vi "总磷总氮公式读取.vi"(8 "error in (no error)":errorcluster caption="错误输入（无错误）", 9 "量程":enum16{"低量程", "高量程"}(ring), 10 "测量模式":enum16{"水样测量", "零点核查", "跨度核查", "标样核查", "加标回收"}(ring), 11 "测量参数":enum16{"COD", "氨氮", "总氮", "总磷"}(ring)) -> (0 "error out":errorcluster caption="错误输出", 3 "公式":cluster{"X^2":dbl, "X":dbl, "b":dbl})   [LabVIEW 2016, in "斯坦道总氮.lvlib"]
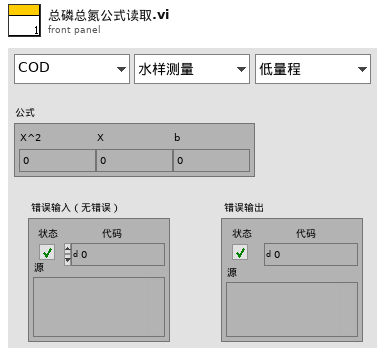
[diagram p1: front panel]
types:
  T1 = cluster{"FLOAT[0]":sgl, "FLOAT[1]":sgl, "FLOAT[2]":sgl}
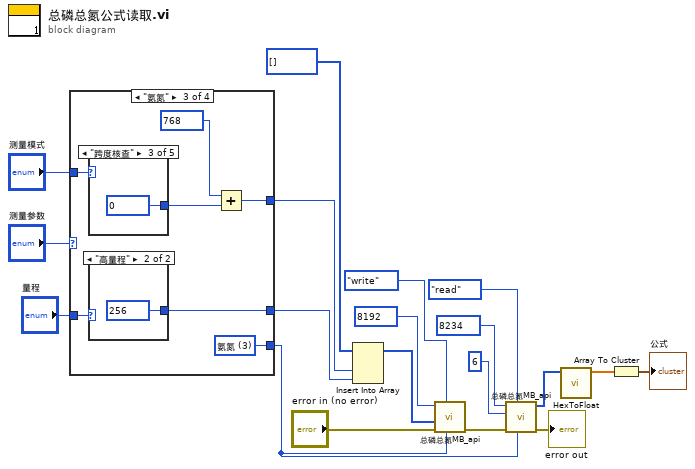
[diagram p0: block diagram]
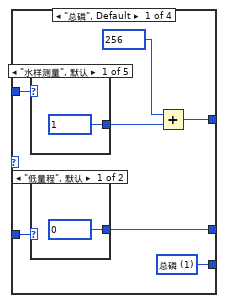
[diagram p2: hidden frame]
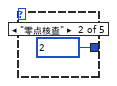
[diagram p3: hidden frame]
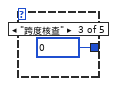
[diagram p4: hidden frame]
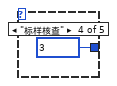
[diagram p5: hidden frame]
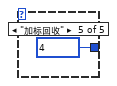
[diagram p6: hidden frame]
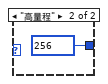
[diagram p7: hidden frame]
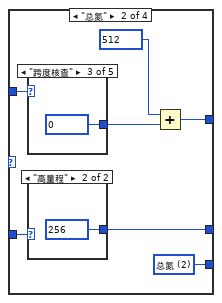
[diagram p8: hidden frame]
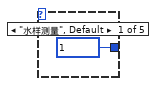
[diagram p9: hidden frame]
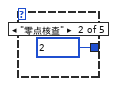
[diagram p10: hidden frame]
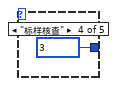
[diagram p11: hidden frame]
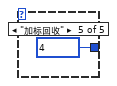
[diagram p12: hidden frame]
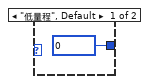
[diagram p13: hidden frame]
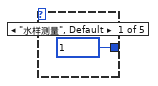
[diagram p14: hidden frame]
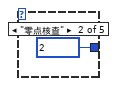
[diagram p15: hidden frame]
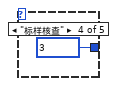
[diagram p16: hidden frame]
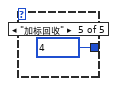
[diagram p17: hidden frame]
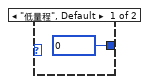
[diagram p18: hidden frame]
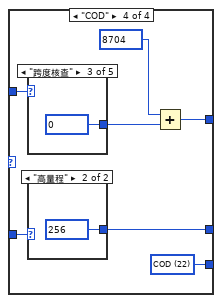
[diagram p19: hidden frame]
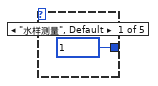
[diagram p20: hidden frame]
diagram:
  n1 = case shown="\"氨氮\"" "测量参数" {
    tunnel: "测量模式" -> [w24 w39 w53 w67]
    tunnel: "量程" -> [w25 w40 w54 w68]
    tunnel: [w26 w34 w48 w62] -> w5
    tunnel: [w20 w35 w49 w63] -> w9
    tunnel: [w23 w38 w52 w66] -> w8
    frame "总磷", Default {
      w26 = u16 1 items=["总磷"=1, "总氮"=2, "氨氮"=3] ("站号")
      n2 = case shown="\"水样测量\", 默认" w24 {
        tunnel: [u16 1 ("starting address") u16 2 ("starting address") u16 0 ("starting address") u16 3 ("starting address") u16 4 ("starting address")] -> w22
        frame "水样测量", Default {
        }
        frame "零点核查" {
        }
        frame "跨度核查" {
        }
        frame "标样核查" {
        }
        frame "加标回收" {
        }
      }
      n3 = case shown="\"低量程\", 默认" w25 {
        tunnel: [u16 0 ("starting address") u16 256 ("starting address")] -> w23
        frame "低量程", Default {
        }
        frame "高量程" {
        }
      }
      n4 = Add(x=u16 256 ("starting address"), y=w22) -> (x+y=w20:u16)
    }
    frame "总氮" {
      w34 = u16 2 items=["总磷"=1, "总氮"=2, "氨氮"=3] ("站号")
      n5 = case shown="\"跨度核查\"" w39 {
        tunnel: [u16 1 ("starting address") u16 2 ("starting address") u16 0 ("starting address") u16 3 ("starting address") u16 4 ("starting address")] -> w37
        frame "水样测量", Default {
        }
        frame "零点核查" {
        }
        frame "跨度核查" {
        }
        frame "标样核查" {
        }
        frame "加标回收" {
        }
      }
      n6 = case shown="\"高量程\"" w40 {
        tunnel: [u16 0 ("starting address") u16 256 ("starting address")] -> w38
        frame "低量程", Default {
        }
        frame "高量程" {
        }
      }
      n7 = Add(x=u16 512 ("starting address"), y=w37) -> (x+y=w35:u16)
    }
    frame "氨氮" {
      w48 = u16 3 items=["总磷"=1, "总氮"=2, "氨氮"=3] ("站号")
      n8 = case shown="\"跨度核查\"" w53 {
        tunnel: [u16 1 ("starting address") u16 2 ("starting address") u16 0 ("starting address") u16 3 ("starting address") u16 4 ("starting address")] -> w51
        frame "水样测量", Default {
        }
        frame "零点核查" {
        }
        frame "跨度核查" {
        }
        frame "标样核查" {
        }
        frame "加标回收" {
        }
      }
      n9 = case shown="\"高量程\"" w54 {
        tunnel: [u16 0 ("starting address") u16 256 ("starting address")] -> w52
        frame "低量程", Default {
        }
        frame "高量程" {
        }
      }
      n10 = Add(x=u16 768 ("starting address"), y=w51) -> (x+y=w49:u16)
    }
    frame "COD" {
      w62 = u16 22 items=["总磷"=1, "总氮"=2, "氨氮"=3, "COD"=22] ("站号")
      n11 = case shown="\"跨度核查\"" w67 {
        tunnel: [u16 1 ("starting address") u16 2 ("starting address") u16 0 ("starting address") u16 3 ("starting address") u16 4 ("starting address")] -> w65
        frame "水样测量", Default {
        }
        frame "零点核查" {
        }
        frame "跨度核查" {
        }
        frame "标样核查" {
        }
        frame "加标回收" {
        }
      }
      n12 = case shown="\"高量程\"" w68 {
        tunnel: [u16 0 ("starting address") u16 256 ("starting address")] -> w66
        frame "低量程", Default {
        }
        frame "高量程" {
        }
      }
      n13 = Add(x=u16 8704 ("starting address"), y=w65) -> (x+y=w63:u16)
    }
  }
  n14 = Insert Into Array(array=u16[] [] ("数组"), new element #1=w9, new element #2=w8) -> (w1:u16[])  [unwired: 1 in]
  n15 = call "总磷总氮MB_api.vi"("Slave ID"=w5, "STEP"=enum16{"open", "read", "write", "close"}."write", "Error in"="error in (no error)", "values"=w1, "starting address"=u16 8192) -> ("error out"=w4:errorcluster)  [unwired: 4 in, 2 out]
  n16 = call "总磷总氮MB_api.vi"("Slave ID"=w5, "STEP"=enum16{"open", "read", "write", "close"}."read", "Error in"=w4, "quantity"=u16 6, "starting address"=u16 8234) -> ("error out"=→"error out":errorcluster, "Registers"=w15:u16[])  [unwired: 4 in, 1 out]
  n17 = call "HexToFloat.vi"("数组"=w15) -> ("FLOAT"=w14:sgl[])  [unwired: 10 in]
  n18 = Array To Cluster(array=w14) -> (cluster=→"公式":T1)
